vi "RFP_Cluster to String_Convert.vi"(3 "Setup String In":string, 4 "Setup Cluster In":T1={"Result files to read"=[], "Template"=path "", "Transpose"=FALSE, "Additional X Values"=[], "Additional Y Values"=[], "Output Filename"=path "", "Create Picture Vi Name"="Intensity plot jpg.vi", "Intensity Plot?"=FALSE, "Multi Ordinate"=[], "Abscissa String"="", "Filter Array"=["", "", "", "", "", ""], "Filter Bins 1 Strings"=[""], "Filter Bins 2 Strings"=[""], "Filters 3 onwards"=[], "nRows"=0} {"Additional Y Values" format="%.2f"; "Additional X Values" format="%.2f"}, 5 "Mode":enum16{"Cluster to String", "String to Cluster"}(ring)) -> (0 "Setup Cluster Out":T1={"Result files to read"=[], "Template"=path "", "Transpose"=FALSE, "Additional X Values"=[], "Additional Y Values"=[], "Output Filename"=path "", "Create Picture Vi Name"="Intensity plot jpg.vi", "Intensity Plot?"=FALSE, "Multi Ordinate"=[], "Abscissa String"="", "Filter Array"=["", "", "", "", "", ""], "Filter Bins 1 Strings"=[""], "Filter Bins 2 Strings"=[""], "Filters 3 onwards"=[], "nRows"=0} {"Additional Y Values" format="%.2f"; "Additional X Values" format="%.2f"}, 1 "Setup String Out":string, 2 "OK?":bool)   [LabVIEW 2022 SP3]
uses:
  Anemometry/Anemometry Sub Vis/Data_plotting_vis/All_Setup.ctl
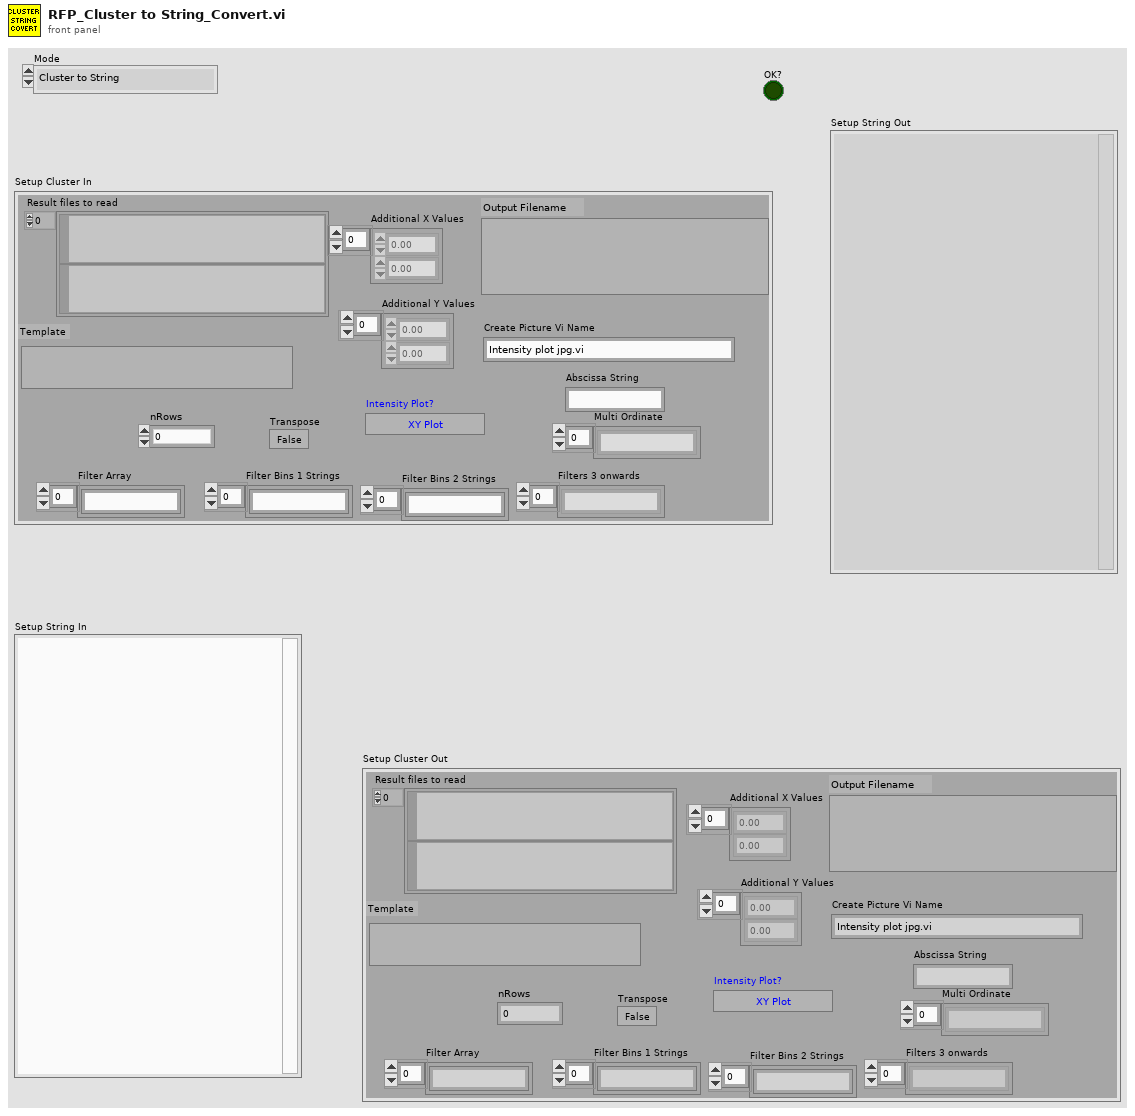
[diagram p1: front panel]
types:
  T1 = typedef "All_Setup.ctl" = cluster{"Result files to read":path[], "Template":path, "Transpose":bool, "Additional X Values":dbl[], "Additional Y Values":dbl[], "Output Filename":path, "Create Picture Vi Name":string, "Intensity Plot?":bool, "Multi Ordinate":string[], "Abscissa String":string, "Filter Array":string[], "Filter Bins 1 Strings":string[], "Filter Bins 2 Strings":string[], "Filters 3 onwards":string[], "nRows":i32}
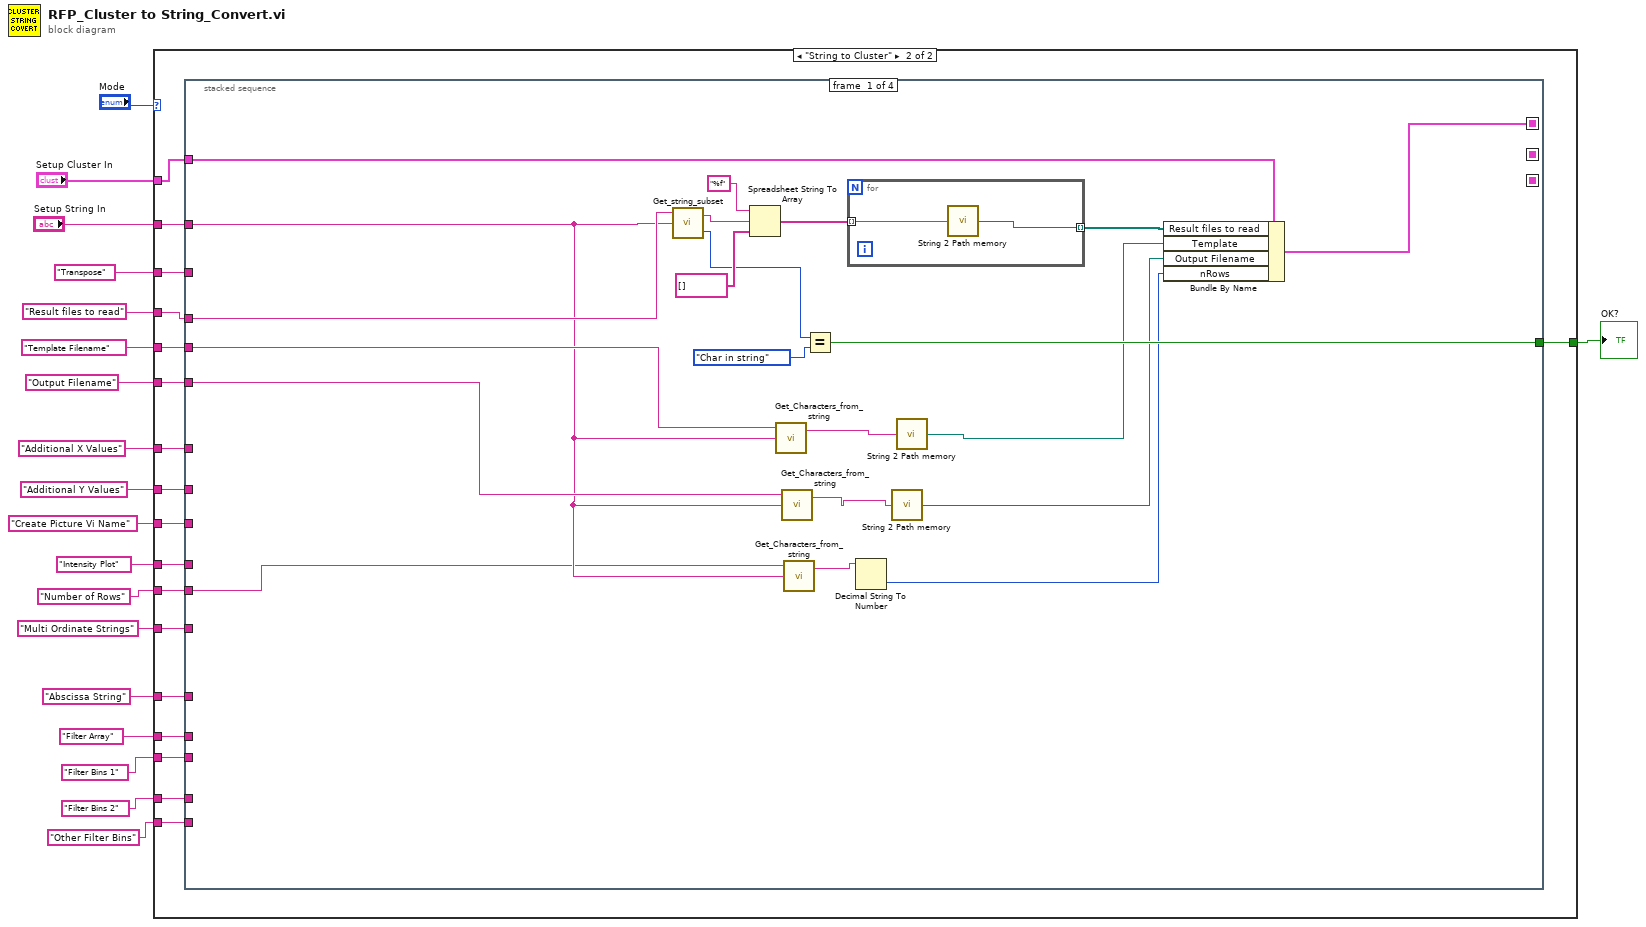
[diagram p0: block diagram]
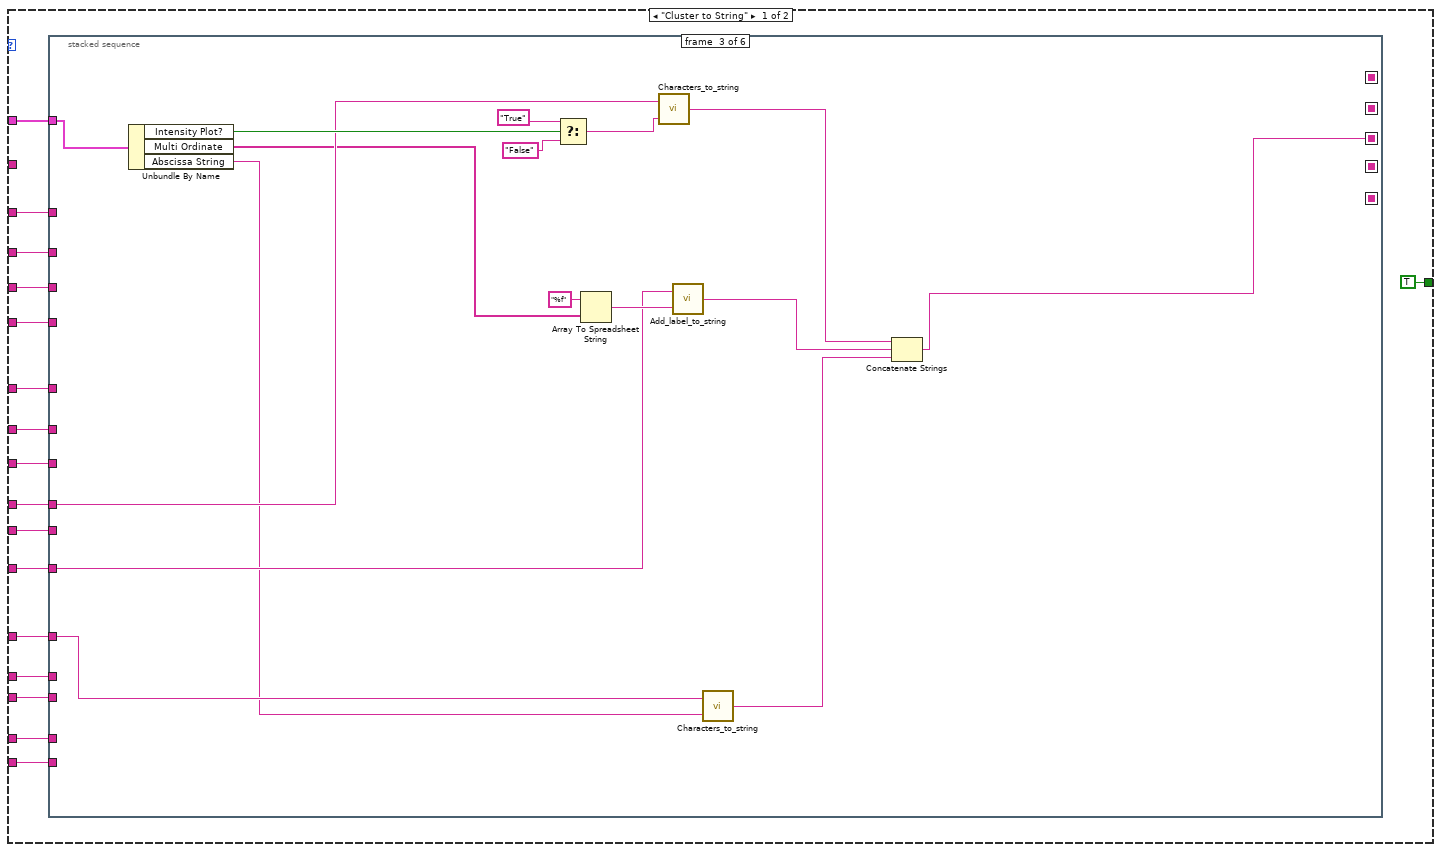
[diagram p2: hidden frame]
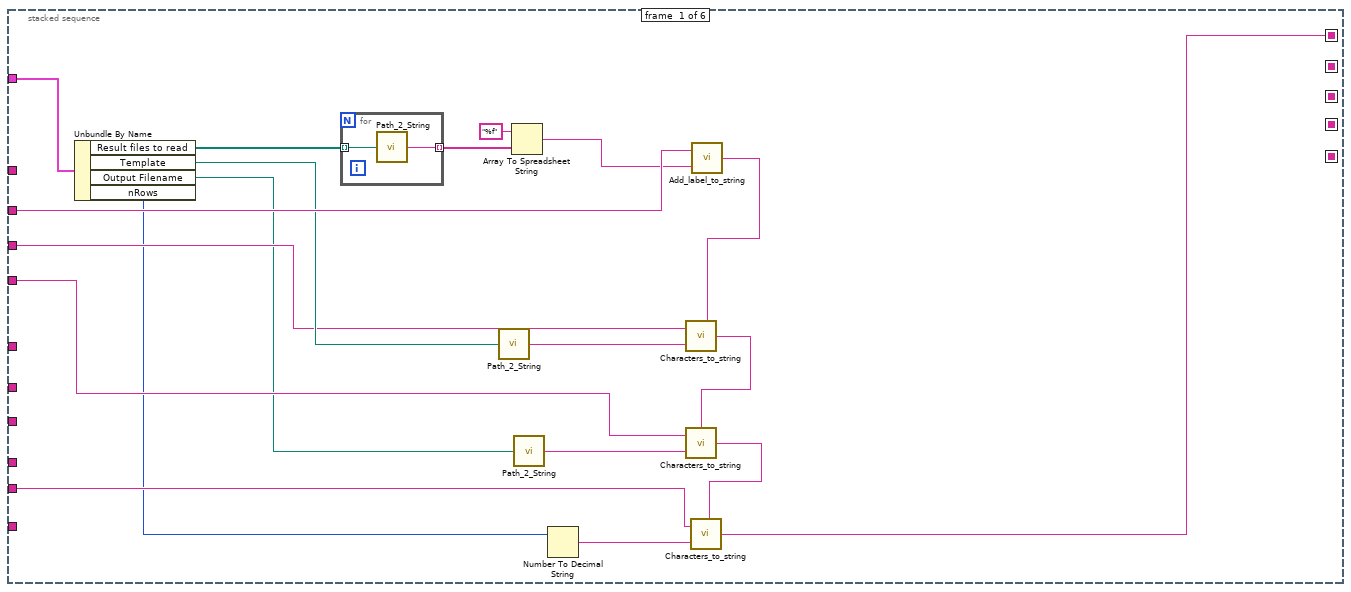
[diagram p3: hidden frame]
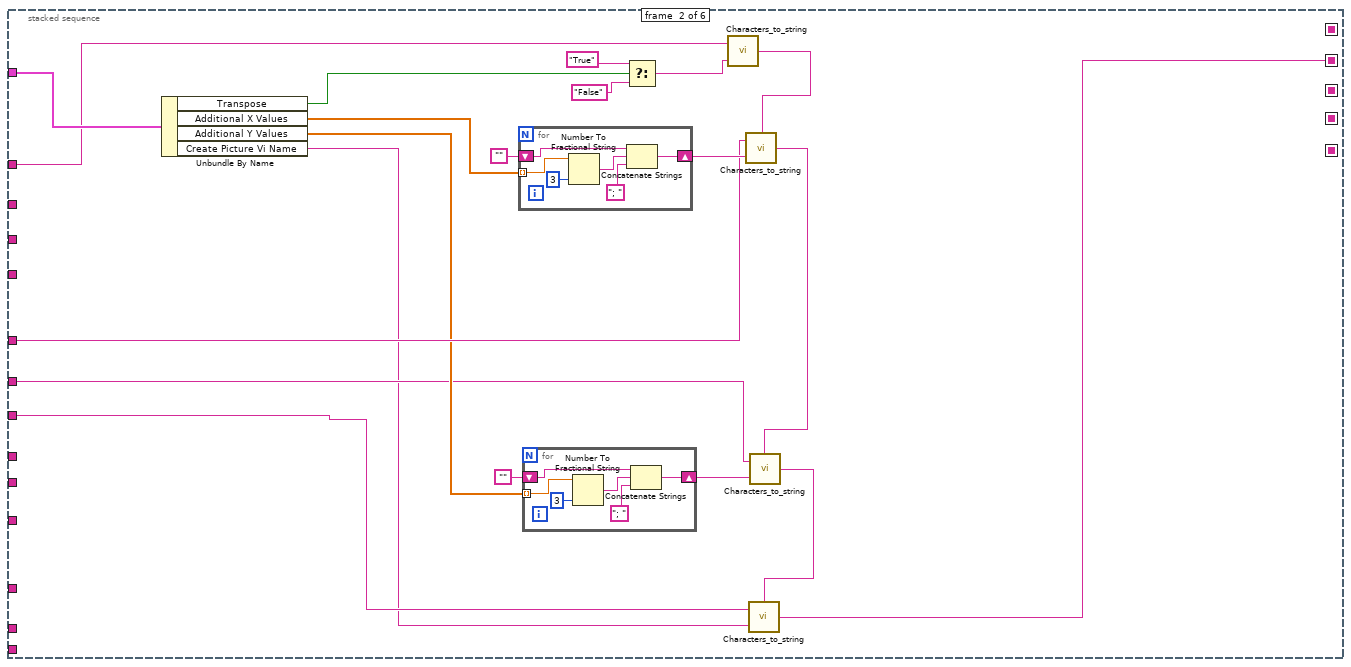
[diagram p4: hidden frame]
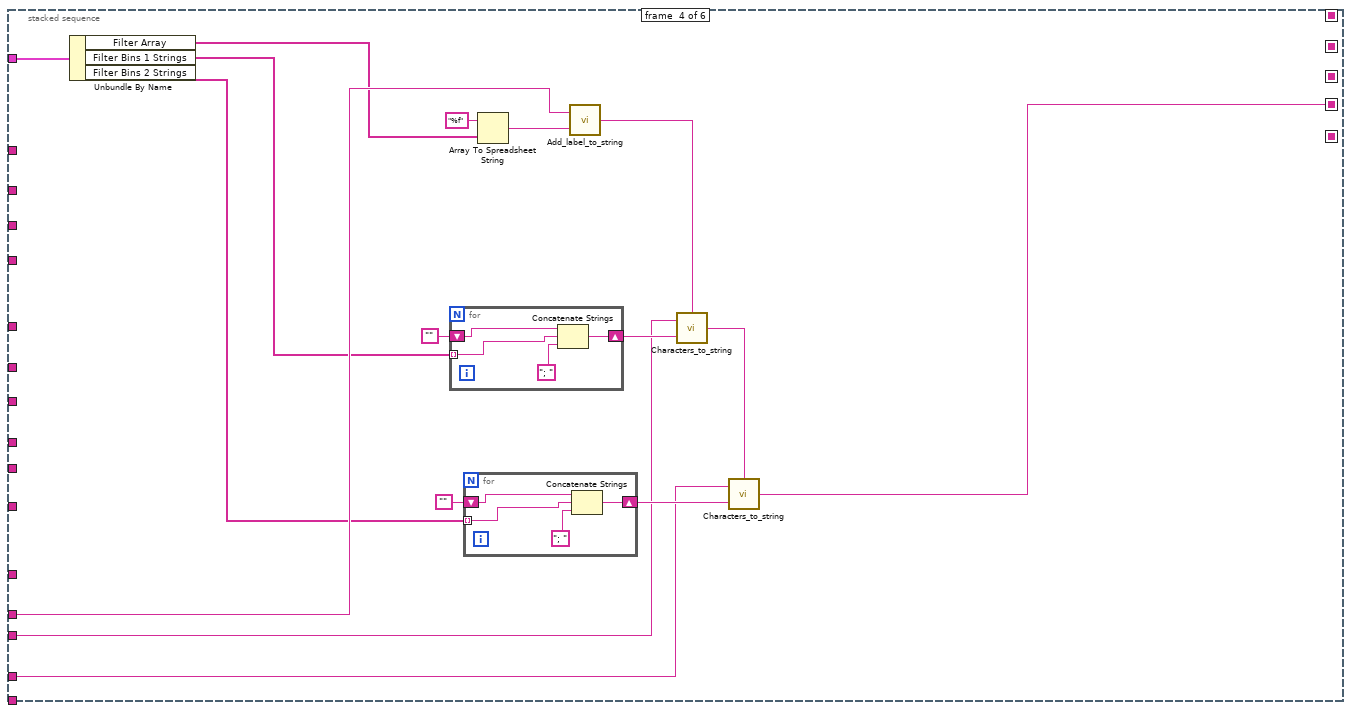
[diagram p5: hidden frame]
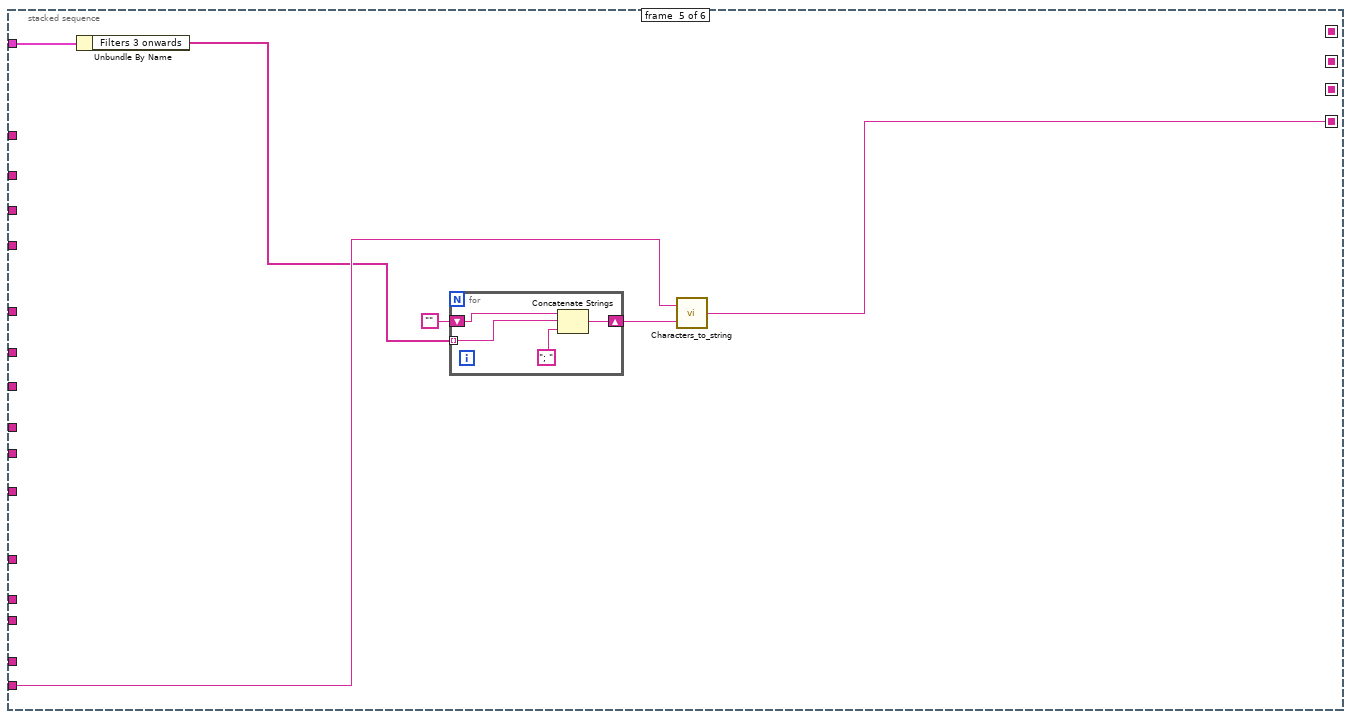
[diagram p6: hidden frame]
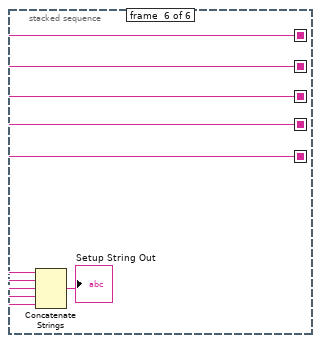
[diagram p7: hidden frame]
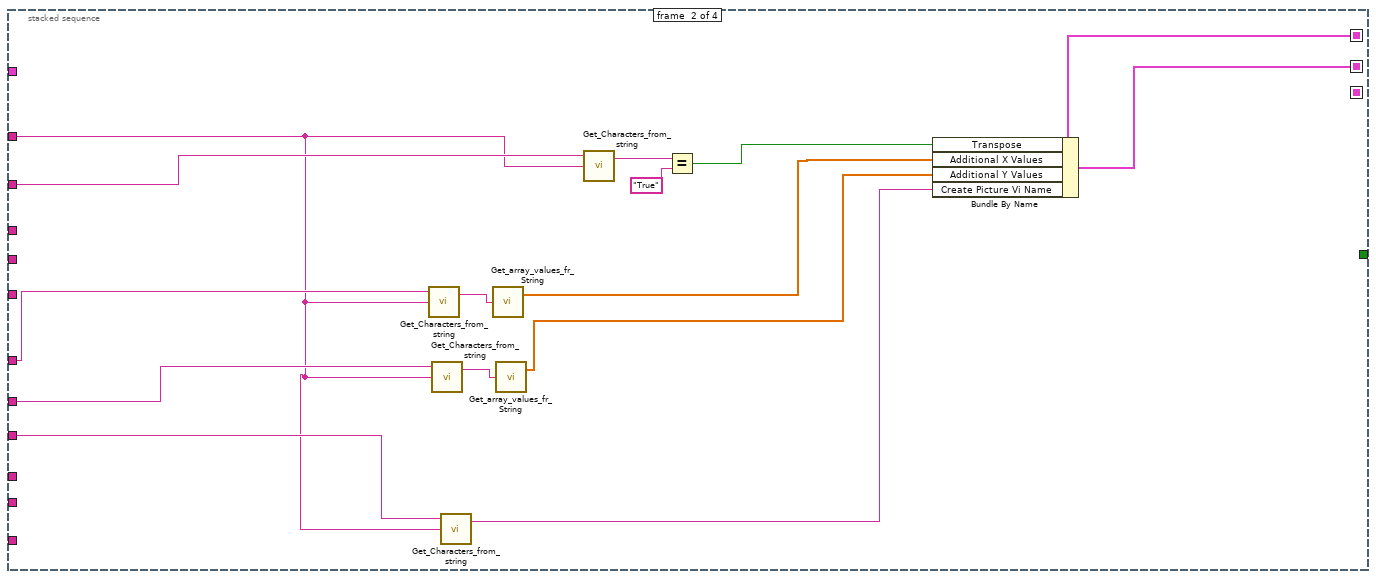
[diagram p8: hidden frame]
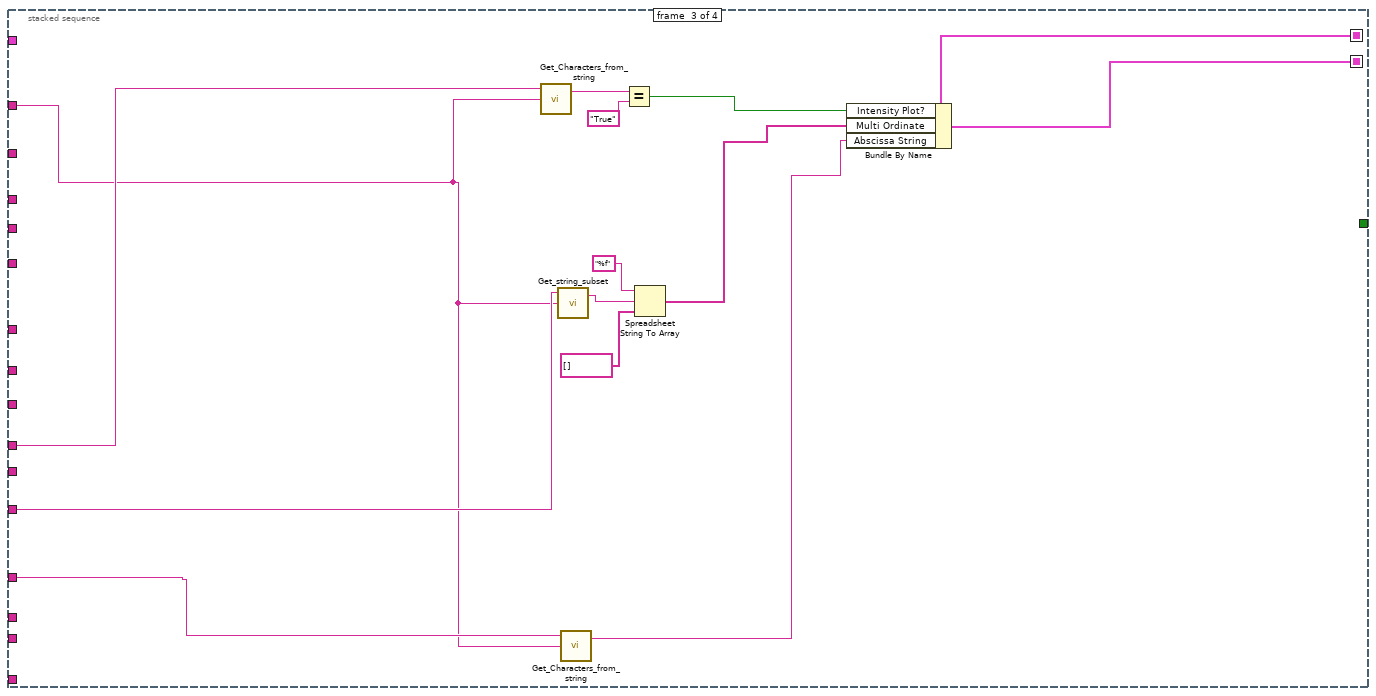
[diagram p9: hidden frame]
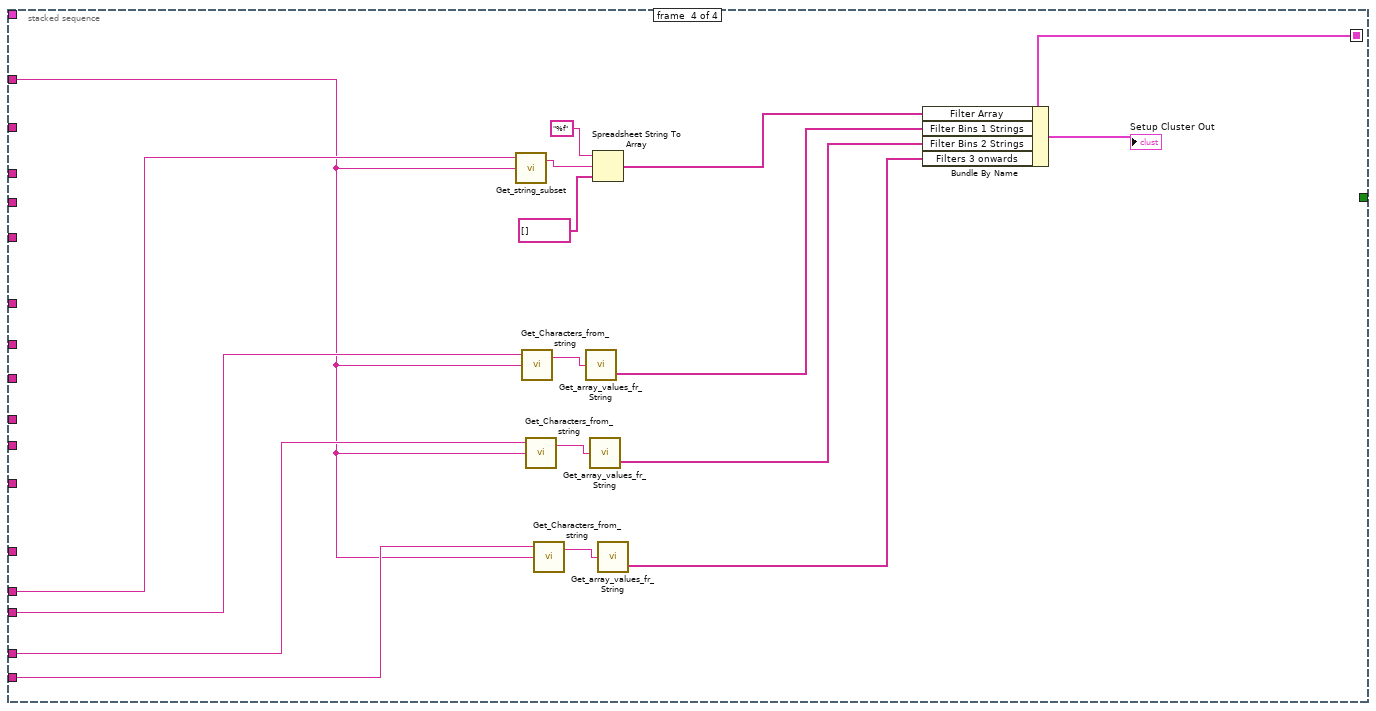
[diagram p10: hidden frame]
diagram:
  n1 = case shown="\"String to Cluster\"" "Mode" {
    tunnel: "Setup Cluster In" -> [w36 w161]
    tunnel: "Result files to read" -> [w35 w162]
    tunnel: "Template Filename" -> [w34 w160]
    tunnel: "Output Filename" -> [w33 w159]
    tunnel: "Additional X Values" -> [w32 w157]
    tunnel: "Transpose" -> [w31 w158]
    tunnel: "Additional Y Values" -> [w30 w156]
    tunnel: "Create Picture Vi Name" -> [w29 w155]
    tunnel: "Intensity Plot" -> [w28 w154]
    tunnel: "Multi Ordinate Strings" -> [w27 w153]
    tunnel: "Abscissa String" -> [w26 w152]
    tunnel: "Filter Array" -> [w25 w151]
    tunnel: "Filter Bins 1" -> [w24 w150]
    tunnel: "Filter Bins 2" -> [w23 w149]
    tunnel: "Setup String In" -> [_ w163]
    tunnel: [TRUE w148] -> w3
    tunnel: "Other Filter Bins" -> [w21 w147]
    tunnel: "Number of Rows" -> [w20 w146]
    frame "Cluster to String" {
      n2 = stacked-sequence {
        seq-local: [w37 _ _ _ _ _] -> [_ _ _ _ _ w145]
        seq-local: [_ w58 _ _ _ _] -> [_ _ _ _ _ w144]
        seq-local: [_ _ w90 _ _ _] -> [_ _ _ _ _ w143]
        seq-local: [_ _ _ w106 _ _] -> [_ _ _ _ _ w142]
        seq-local: [_ _ _ _ w131 _] -> [_ _ _ _ _ w140]
        tunnel: w36 -> [w44 w77 w105 w121 w135 _]
        tunnel: w35 -> [w52 _ _ _ _ _]
        tunnel: w34 -> [w47 _ _ _ _ _]
        tunnel: w33 -> [w46 _ _ _ _ _]
        tunnel: w32 -> [_ w73 _ _ _ _]
        tunnel: w31 -> [_ w72 _ _ _ _]
        tunnel: w30 -> [_ w64 _ _ _ _]
        tunnel: w29 -> [_ w63 _ _ _ _]
        tunnel: w28 -> [_ _ w100 _ _ _]
        tunnel: w27 -> [_ _ w96 _ _ _]
        tunnel: w26 -> [_ _ w95 _ _ _]
        tunnel: w25 -> [_ _ _ w118 _ _]
        tunnel: w24 -> [_ _ _ w111 _ _]
        tunnel: w23 -> [_ _ _ w110 _ _]
        tunnel: w21 -> [_ _ _ _ w132 _]
        tunnel: w20 -> [w43 _ _ _ _ _]
        frame #0 {
          n3 = Unbundle By Name(w44) -> ("Result files to read"=w55:path[], "Template"=w50:path, "Output Filename"=w45:path, "nRows"=w42:i32)
          n4 = for {
            tunnel: w55 -> [w57] mode=indexing
            tunnel: [w56] -> w54 mode=indexing
            n5 = call "Path_2_String.vi"("Real Path"=w57) -> ("Path String"=w56:string)
          }
          n6 = call "Path_2_String.vi"("Real Path"=w50) -> ("Path String"=w49:string)
          n7 = Array To Spreadsheet String(array=w54, 3:"%f" ("format string")) -> (spreadsheet string=w51:string)  [unwired: 1 in]
          n8 = call "Path_2_String.vi"("Real Path"=w45) -> ("Path String"=w48:string)
          n9 = Number To Decimal String(number=w42) -> (decimal integer string=w41:string)  [unwired: 1 in]
          n10 = call "Add_label_to_string.vi"("String to write"=w51, "File Label"=w52) -> ("Output string"=w40:string)
          n11 = call "Characters_to_string.vi"("stringIn"=w40, "Characters to write"=w49, "Label for characters"=w47) -> ("Output string"=w39:string)
          n12 = call "Characters_to_string.vi"("stringIn"=w39, "Characters to write"=w48, "Label for characters"=w46) -> ("Output string"=w38:string)
          n13 = call "Characters_to_string.vi"("stringIn"=w38, "Characters to write"=w41, "Label for characters"=w43) -> ("Output string"=w37:string)
        }
        frame #1 {
          n14 = Unbundle By Name(w77) -> ("Transpose"=w71:bool, "Additional X Values"=w74:dbl[], "Additional Y Values"=w65:dbl[], "Create Picture Vi Name"=w62:string)
          n15 = for {
            shift-right: [w85] -> w75
            shift-left: "" -> [w88]
            tunnel: w74 -> [w89] mode=indexing
            n16 = Number To Fractional String(number=w89, precision (6)=i16 3) -> (F-format string=w87:string)  [unwired: 2 in]
            n17 = Concatenate Strings(w88, w87, "; ") -> (w85:string)
          }
          n18 = for {
            shift-right: [w79] -> w67
            shift-left: "" -> [w82]
            tunnel: w65 -> [w83] mode=indexing
            n19 = Number To Fractional String(number=w83, precision (6)=i16 3) -> (F-format string=w81:string)  [unwired: 2 in]
            n20 = Concatenate Strings(w82, w81, "; ") -> (w79:string)
          }
          n21 = Select(t="True", s=w71, f="False") -> (s? t:f=w68:string)
          n22 = call "Characters_to_string.vi"("Characters to write"=w68, "Label for characters"=w72) -> ("Output string"=w61:string)  [unwired: 1 in]
          n23 = call "Characters_to_string.vi"("stringIn"=w61, "Characters to write"=w75, "Label for characters"=w73) -> ("Output string"=w60:string)
          n24 = call "Characters_to_string.vi"("stringIn"=w60, "Characters to write"=w67, "Label for characters"=w64) -> ("Output string"=w59:string)
          n25 = call "Characters_to_string.vi"("stringIn"=w59, "Characters to write"=w62, "Label for characters"=w63) -> ("Output string"=w58:string)
        }
        frame #2 {
          n26 = Unbundle By Name(w105) -> ("Intensity Plot?"=w101:bool, "Multi Ordinate"=w98:string[], "Abscissa String"=w94:string)
          n27 = Select(t="True", s=w101, f="False") -> (s? t:f=w102:string)
          n28 = Array To Spreadsheet String(array=w98, 3:"%f" ("format string")) -> (spreadsheet string=w97:string)  [unwired: 1 in]
          n29 = call "Characters_to_string.vi"("Characters to write"=w102, "Label for characters"=w100) -> ("Output string"=w93:string)  [unwired: 1 in]
          n30 = call "Add_label_to_string.vi"("String to write"=w97, "File Label"=w96) -> ("Output string"=w92:string)
          n31 = call "Characters_to_string.vi"("Characters to write"=w94, "Label for characters"=w95) -> ("Output string"=w91:string)  [unwired: 1 in]
          n32 = Concatenate Strings(w93, w92, w91) -> (w90:string)
        }
        frame #3 {
          n33 = Unbundle By Name(w121) -> ("Filter Array"=w117:string[], "Filter Bins 1 Strings"=w114:string[], "Filter Bins 2 Strings"=w109:string[])
          n34 = for {
            shift-right: [w127] -> w116
            shift-left: "" -> [w129]
            tunnel: w114 -> [w126] mode=indexing
            n35 = Concatenate Strings(w129, w126, "; ") -> (w127:string)
          }
          n36 = for {
            shift-right: [w123] -> w112
            shift-left: "" -> [w125]
            tunnel: w109 -> [w122] mode=indexing
            n37 = Concatenate Strings(w125, w122, "; ") -> (w123:string)
          }
          n38 = Array To Spreadsheet String(array=w117, 3:"%f" ("format string")) -> (spreadsheet string=w119:string)  [unwired: 1 in]
          n39 = call "Add_label_to_string.vi"("String to write"=w119, "File Label"=w118) -> ("Output string"=w108:string)
          n40 = call "Characters_to_string.vi"("stringIn"=w108, "Characters to write"=w116, "Label for characters"=w111) -> ("Output string"=w107:string)
          n41 = call "Characters_to_string.vi"("stringIn"=w107, "Characters to write"=w112, "Label for characters"=w110) -> ("Output string"=w106:string)
        }
        frame #4 {
          n42 = Unbundle By Name(w135) -> ("Filters 3 onwards"=w130:string[])
          n43 = for {
            shift-right: [w137] -> w134
            shift-left: "" -> [w139]
            tunnel: w130 -> [w136] mode=indexing
            n44 = Concatenate Strings(w139, w136, "; ") -> (w137:string)
          }
          n45 = call "Characters_to_string.vi"("Characters to write"=w134, "Label for characters"=w132) -> ("Output string"=w131:string)  [unwired: 1 in]
        }
        frame #5 {
          n46 = Concatenate Strings(w145, w144, w143, w142, w140) -> (→"Setup String Out":string)
        }
      }
    }
    frame "String to Cluster" {
      n47 = stacked-sequence {
        seq-local: [w172 _ _ _] -> [_ w201 _ _]
        seq-local: [_ w187 _ _] -> [_ _ w215 _]
        seq-local: [_ _ w202 _] -> [_ _ _ w232]
        tunnel: w163 -> [w171 w189 w203 w219]
        tunnel: w162 -> [w184 _ _ _]
        tunnel: w161 -> [w180 _ _ _]
        tunnel: w160 -> [w177 _ _ _]
        tunnel: w159 -> [w176 _ _ _]
        tunnel: w158 -> [_ w200 _ _]
        tunnel: w157 -> [_ w195 _ _]
        tunnel: w156 -> [_ w193 _ _]
        tunnel: w155 -> [_ w190 _ _]
        tunnel: w154 -> [_ _ w212 _]
        tunnel: w153 -> [_ _ w207 _]
        tunnel: w152 -> [_ _ w204 _]
        tunnel: w151 -> [_ _ _ w228]
        tunnel: w150 -> [_ _ _ w225]
        tunnel: w149 -> [_ _ _ w223]
        tunnel: [w173 _ _ _] -> w148
        tunnel: w147 -> [_ _ _ w220]
        tunnel: w146 -> [w170 _ _ _]
        frame #0 {
          n48 = call "Get_string_subset.vi"("String to split"=w171, "File Label"=w184) -> ("Status"=w174:enum16{"Char in string", "Char not in string"}, "Output string"=w183:string)  [unwired: 2 in]
          n49 = Spreadsheet String To Array(format string="%f", spreadsheet string=w183, array type (2D Dbl)=string[] []) -> (array=w179:string[])  [unwired: 1 in]
          n50 = call "Get_Characters_from_string.vi"("Input string"=w171, "Variable name"=w177) -> ("Value"=w167:string)  [unwired: 1 in, 1 out]
          n51 = call "Get_Characters_from_string.vi"("Input string"=w171, "Variable name"=w176) -> ("Value"=w165:string)  [unwired: 1 in, 1 out]
          n52 = call "Get_Characters_from_string.vi"("Input string"=w171, "Variable name"=w170) -> ("Value"=w169:string)  [unwired: 1 in, 1 out]
          n53 = Equal?(x=w174, y=enum16{"Char in string", "Char not in string"}."Char in string" ("Status")) -> (x = y?=w173:bool)
          n54 = for {
            tunnel: w179 -> [w186] mode=indexing
            tunnel: [w185] -> w178 mode=indexing
            n55 = call "String 2 Path memory.vi"("Input String"=w186) -> ("path"=w185:path)  [unwired: 1 in]
          }
          n56 = Decimal String To Number(string=w169) -> (number=w168:i32)  [unwired: 2 in, 1 out]
          n57 = call "String 2 Path memory.vi"("Input String"=w165) -> ("path"=w164:path)  [unwired: 1 in]
          n58 = call "String 2 Path memory.vi"("Input String"=w167) -> ("path"=w166:path)  [unwired: 1 in]
          n59 = Bundle By Name(cluster=w180, "Result files to read"=w178, "Template"=w166, "Output Filename"=w164, "nRows"=w168) -> (w172:T1)
        }
        frame #1 {
          n60 = call "Get_Characters_from_string.vi"("Input string"=w189, "Variable name"=w195) -> ("Value"=w196:string)  [unwired: 1 in, 1 out]
          n61 = call "Get_Characters_from_string.vi"("Input string"=w189, "Variable name"=w193) -> ("Value"=w194:string)  [unwired: 1 in, 1 out]
          n62 = call "Get_Characters_from_string.vi"("Input string"=w189, "Variable name"=w190) -> ("Value"=w188:string)  [unwired: 1 in, 1 out]
          n63 = call "Get_array_values_fr_String.vi"("String Value"=w196) -> ("Numeric Array"=w192:dbl[])  [unwired: 1 out]
          n64 = call "Get_array_values_fr_String.vi"("String Value"=w194) -> ("Numeric Array"=w191:dbl[])  [unwired: 1 out]
          n65 = call "Get_Characters_from_string.vi"("Input string"=w189, "Variable name"=w200) -> ("Value"=w199:string)  [unwired: 1 in, 1 out]
          n66 = Equal?(x=w199, y="True") -> (x = y?=w197:bool)
          n67 = Bundle By Name(cluster=w201, "Transpose"=w197, "Additional X Values"=w192, "Additional Y Values"=w191, "Create Picture Vi Name"=w188) -> (w187:T1)
        }
        frame #2 {
          n68 = call "Get_Characters_from_string.vi"("Input string"=w203, "Variable name"=w212) -> ("Value"=w214:string)  [unwired: 1 in, 1 out]
          n69 = call "Get_string_subset.vi"("String to split"=w203, "File Label"=w207) -> ("Output string"=w210:string)  [unwired: 2 in, 1 out]
          n70 = call "Get_Characters_from_string.vi"("Input string"=w203, "Variable name"=w204) -> ("Value"=w205:string)  [unwired: 1 in, 1 out]
          n71 = Equal?(x=w214, y="True") -> (x = y?=w211:bool)
          n72 = Spreadsheet String To Array(format string="%f", spreadsheet string=w210, array type (2D Dbl)=string[] []) -> (array=w206:string[])  [unwired: 1 in]
          n73 = Bundle By Name(cluster=w215, "Intensity Plot?"=w211, "Multi Ordinate"=w206, "Abscissa String"=w205) -> (w202:T1)
        }
        frame #3 {
          n74 = call "Get_string_subset.vi"("String to split"=w219, "File Label"=w228) -> ("Output string"=w231:string)  [unwired: 2 in, 1 out]
          n75 = call "Get_Characters_from_string.vi"("Input string"=w219, "Variable name"=w225) -> ("Value"=w226:string)  [unwired: 1 in, 1 out]
          n76 = call "Get_Characters_from_string.vi"("Input string"=w219, "Variable name"=w223) -> ("Value"=w224:string)  [unwired: 1 in, 1 out]
          n77 = call "Get_Characters_from_string.vi"("Input string"=w219, "Variable name"=w220) -> ("Value"=w221:string)  [unwired: 1 in, 1 out]
          n78 = call "Get_array_values_fr_String.vi"("String Value"=w226) -> ("String array"=w218:string[])  [unwired: 1 out]
          n79 = call "Get_array_values_fr_String.vi"("String Value"=w224) -> ("String array"=w217:string[])  [unwired: 1 out]
          n80 = Spreadsheet String To Array(format string="%f", spreadsheet string=w231, array type (2D Dbl)=string[] []) -> (array=w227:string[])  [unwired: 1 in]
          n81 = call "Get_array_values_fr_String.vi"("String Value"=w221) -> ("String array"=w216:string[])  [unwired: 1 out]
          n82 = Bundle By Name(cluster=w232, "Filter Array"=w227, "Filter Bins 1 Strings"=w218, "Filter Bins 2 Strings"=w217, "Filters 3 onwards"=w216) -> (→"Setup Cluster Out":T1)
        }
      }
    }
  }
  "OK?" <- w3
